vi "Convert String to Double.vi"(8 "Input String":string, 10 "Conversion Type (6)":i32=6, 11 "String Offset (0)":i32) -> (3 "Converted Output":dbl format="%#.3e")   [LabVIEW 2014, in "Fluke 190 Series II.lvlib"]
doc: "Converts a hex character string into a double value."
uses:
  Fluke 190 Series II.lvlib
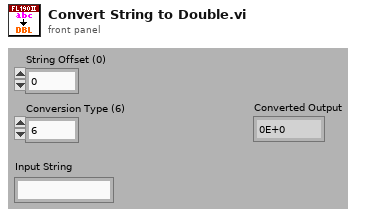
[diagram p1: front panel]
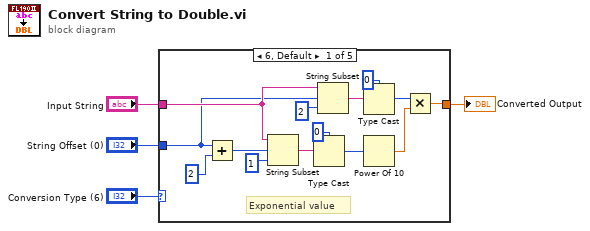
[diagram p0: block diagram]
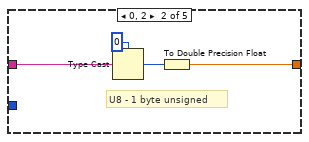
[diagram p2: hidden frame]
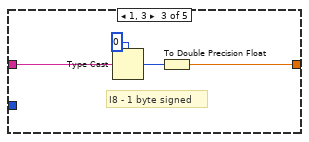
[diagram p3: hidden frame]
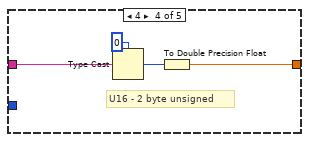
[diagram p4: hidden frame]
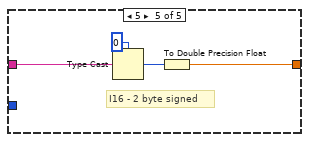
[diagram p5: hidden frame]
diagram:
  n1 = case shown="6, Default" "Conversion Type (6)" {
    tunnel: "Input String" -> [w7 w21 w25 w29 w33]
    tunnel: [w6 w19 w23 w27 w31] -> w2
    tunnel: "String Offset (0)" -> [w5 _ _ _ _]
    frame 6, Default {
      # "Exponential value"
      n2 = Add(x=w5, y=u32 2 ("x")) -> (x+y=w15:u32)
      n3 = String Subset(string=w7, offset (0)=w15, length (rest)=1 ("length (rest)")) -> (substring=w11:string)
      n4 = Type Cast(type=i8 0, x=w11) -> (*(type *) &x=w10:i8)
      n5 = String Subset(string=w7, offset (0)=w5, length (rest)=2 ("length (rest)")) -> (substring=w14:string)
      n6 = Type Cast(type=i16 0, x=w14) -> (*(type *) &x=w9:i16)
      n7 = Power Of 10(x=w10) -> (10^x=w8:dbl)
      n8 = Multiply(x=w9, y=w8) -> (x*y=w6:dbl)
    }
    frame 0, 2 {
      # "U8 - 1 byte unsigned"
      n9 = Type Cast(type=u8 0, x=w21) -> (*(type *) &x=w20:u8)
      n10 = To Double Precision Float(number=w20) -> (double precision float=w19:dbl)
    }
    frame 1, 3 {
      # "I8 - 1 byte signed"
      n11 = Type Cast(type=i8 0, x=w25) -> (*(type *) &x=w24:i8)
      n12 = To Double Precision Float(number=w24) -> (double precision float=w23:dbl)
    }
    frame 4 {
      # "U16 - 2 byte unsigned"
      n13 = Type Cast(type=u16 0, x=w29) -> (*(type *) &x=w28:u16)
      n14 = To Double Precision Float(number=w28) -> (double precision float=w27:dbl)
    }
    frame 5 {
      # "I16 - 2 byte signed"
      n15 = Type Cast(type=i16 0, x=w33) -> (*(type *) &x=w32:i16)
      n16 = To Double Precision Float(number=w32) -> (double precision float=w31:dbl)
    }
  }
  "Converted Output" <- w2
